vi "irisMove.vi"(1 "size (um)":dbl) -> ()   [LabVIEW 2017]
uses:
  globalDevices.vi
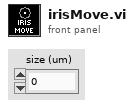
[diagram p1: front panel]
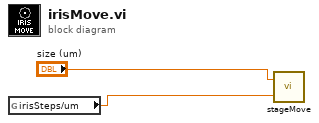
[diagram p0: block diagram]
diagram:
  n1 = global read "globalDevices.vi" "irisSteps/um"() -> (w2:dbl)
  n2 = call "stageMove.vi"("counts/um"=w2, "position (um)"="size (um)") -> ()  [unwired: 2 out]
